vi "mod_Burst Detector.vi"(0 "IQ data (complex) in":cluster{"t0":dbl, "dt":dbl, "Y":cdb[]}={"t0"=0.0, "dt"=1.0, "Y"=[]} {"Y" format="%.2f"; "dt" format="%.2f"; "t0" format="%.2f"}, 1 "RC":dbl=0.001, 5 "Rise Trigger Specs":T2, 7 "Fall Trigger Specs":T1, 9 "Detection":enum16{"Simple", "Advanced"}(ring), 11 "error in (no error)":errorcluster, 12 "SC":dbl=0.0002, 13 "reset ? (T)":bool) -> (4 "Signal Envelope":waveform(dbl)(graph), 6 "Bursts Detected?":bool, 8 "Bursts Found":cluster{"Start Index":dbl, "Stop Index":dbl}[](array[cluster]), 10 "Number of Bursts":i32, 15 "error out":errorcluster)   [LabVIEW 2020, in "niDMT.lvlib"]
doc: "This utility detects multiple bursts. You can adjust the Discharge Time Constant (RC) and Charge Time Constant (SC) for detecting burst with short dead time between them. A lower value of RC implies fast discharging. For bursts very closely space, the discharging in the burst detector should happen fast so that falling slope is detected. Similarly SC can adjusted to detect rising between closely spaced bursts. Typically, the default values should work fine."
uses:
  <vilib>/addons/Modulation/niDMT.lvlib
  <vilib>/Analysis/baseanly.llb/Mean (DBL).vi
  <vilib>/measure/mamon.llb/Trigger Detection for 1 Channel (obs).vi
  <vilib>/Waveform/WDTOps.llb/WDT Get Waveform Subset DBL (LV80).vi
  <vilib>/addons/Modulation/niAMT.lvlib
  <vilib>/Analysis/NI_AALBase.lvlib
  <vilib>/measure/NI_MAPro.lvlib
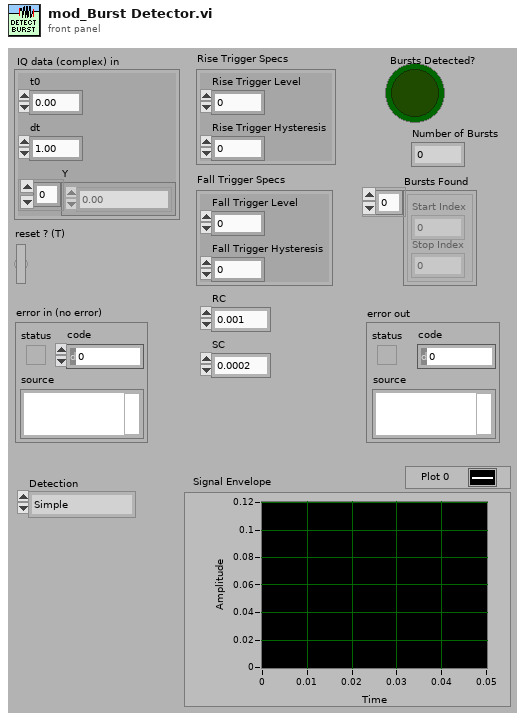
[diagram p1: front panel]
types:
  T1 = cluster{"Fall Trigger Level":dbl, "Fall Trigger Hysteresis":dbl}
  T2 = cluster{"Rise Trigger Level":dbl, "Rise Trigger Hysteresis":dbl}
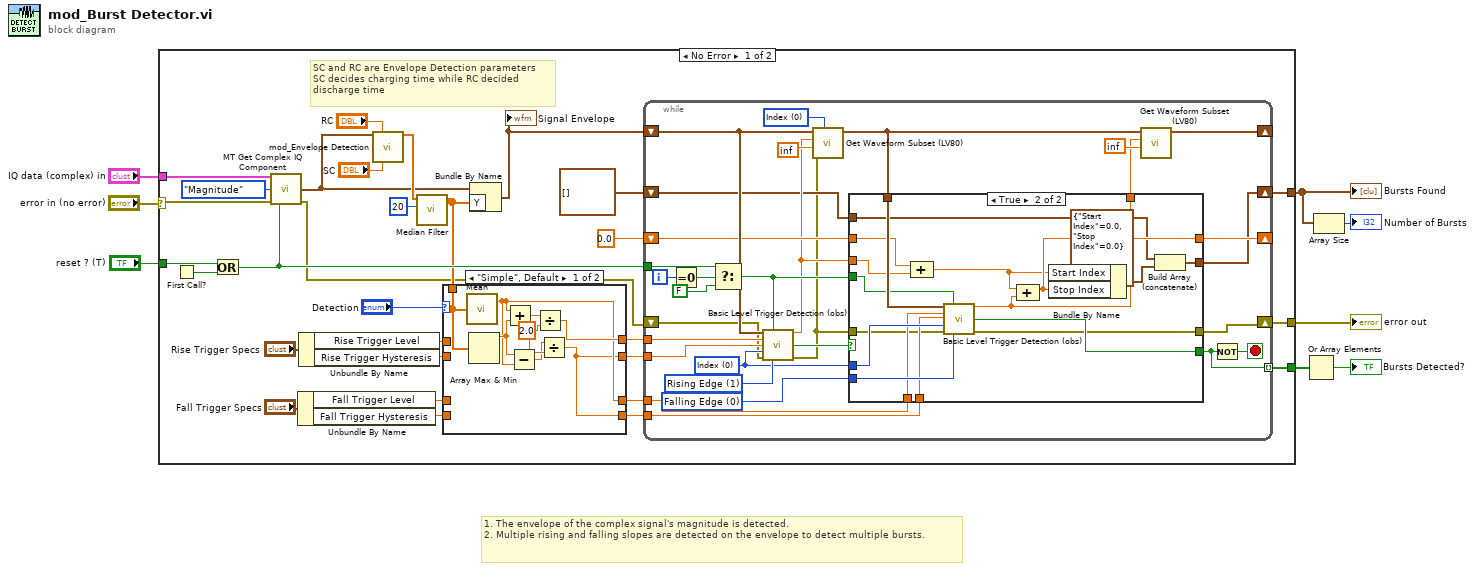
[diagram p0: block diagram]
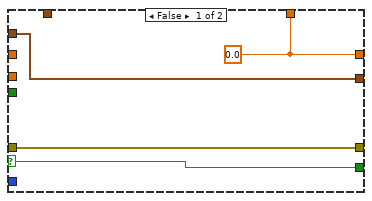
[diagram p3: hidden frame]
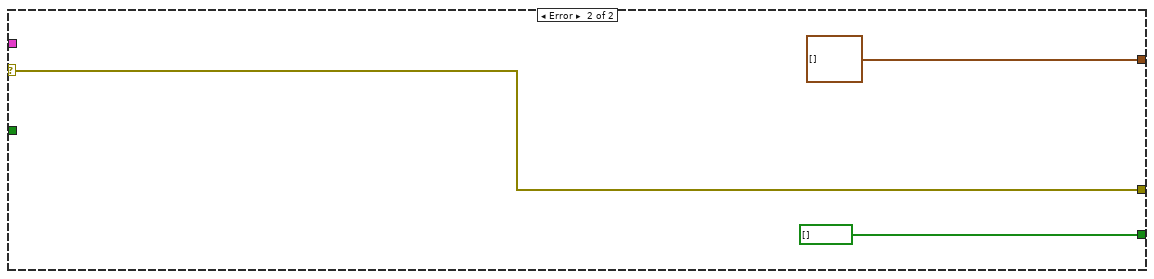
[diagram p4: hidden frame]
diagram:
  # "1. The envelope of the complex signal's magnitude is detected. \n2. Multiple rising and falling slopes are detected on the envelope to detect multiple bursts."
  n1 = case shown="No Error" "error in (no error)" {
    selector: "error in (no error)" -> [w37 w105]
    tunnel: "IQ data (complex) in" -> [w38 _]
    tunnel: "reset ? (T)" -> [w34 _]
    tunnel: [w24 cluster{"Start Index":dbl, "Stop Index":dbl}[] []] -> w2
    tunnel: [w22 bool[] []] -> w5
    tunnel: [w21 w105] -> w3
    frame No Error {
      # "SC and RC are Envelope Detection parameters\nSC decides charging time while RC decided \ndischarge time"
      n2 = First Call?() -> (First Call?: T/F=w35:bool)
      n3 = Or(x=w34, y=w35) -> (x .or. y?=w28:bool)
      n4 = call <vilib>:"MT Get Complex IQ Component.vi"("IQ data (complex) in"=w38, "reset? (F)"=w28, "component choice"=enum16{"I", "Q", "Magnitude", "Phase"}."Magnitude", "error in (no error)"=w37) -> ("CE component"=w29:waveform(dbl), "error out"=w9:errorcluster)  [unwired: 10 out]
      n5 = Unbundle By Name("Fall Trigger Specs") -> ("Fall Trigger Level"=w13:dbl, "Fall Trigger Hysteresis"=w11:dbl)
      n6 = Unbundle By Name("Rise Trigger Specs") -> ("Rise Trigger Level"=w15:dbl, "Rise Trigger Hysteresis"=w14:dbl)
      n7 = call <vilib>:"mod_Envelope Detection.vi"("input data"=w29, "RC"="RC", "SC"="SC") -> ("QP Output"=w31:dbl[])  [unwired: 12 out]
      n8 = call <vilib>:"Median Filter.vi"("left rank"=20 ("rank"), "X"=w31) -> ("Filtered X"=w19:dbl[])  [unwired: 1 in, 8 out]
      n9 = case shown="\"Simple\", Default" "Detection" {
        tunnel: w19 -> [w46 _]
        tunnel: [w40 w48] -> w18
        tunnel: [w39 w49] -> w17
        tunnel: [w44 w50] -> w16
        tunnel: w15 -> [_ w50]
        tunnel: w14 -> [_ w49]
        tunnel: w13 -> [_ w48]
        tunnel: [w39 w47] -> w12
        tunnel: w11 -> [_ w47]
        frame "Simple", Default {
          w42 = 2.0 ("y")
          n10 = call-poly <vilib>:"Mean.vi"("X"=w46) -> ("mean"=w40:dbl)  [unwired: 1 out]
          n11 = Array Max & Min(array=w46) -> (max value=w43:dbl)  [unwired: 3 out]
          n12 = Add(x=w40, y=w43) -> (x+y=w45:dbl)
          n13 = Subtract(x=w43, y=w40) -> (x-y=w41:dbl)
          n14 = Divide(x=w45, y=w42) -> (x/y=w44:dbl)
          n15 = Divide(x=w41, y=w42) -> (x/y=w39:dbl)
        }
        frame "Advanced" {
        }
      }
      n16 = Bundle By Name(cluster=w29, "Y"=w19) -> (w20:waveform(dbl))
      "Signal Envelope" <- w20
      n17 = while {
        shift-right: [w60] -> _
        shift-left: w20 -> [w72]
        tunnel: w28 -> [w78]
        tunnel: w16 -> [w77]
        tunnel: w17 -> [w76]
        tunnel: w18 -> [w68]
        tunnel: w12 -> [w67]
        shift-right: [w59] -> _
        shift-left: 0.0 -> [w62]
        shift-right: [w58] -> w24
        shift-left: cluster{"Start Index":dbl, "Stop Index":dbl}[] [] -> [w57]
        tunnel: [w55] -> w22 mode=indexing
        shift-right: [w51] -> w21
        shift-left: w9 -> [w53]
        i -> [w80]
        stop <- w56 stop-if-true
        w66 = u16 0 items=["Index", "Relative Time"] ("Mode")
        w69 = u16 0 items=["Falling Edge", "Rising Edge"] ("slope")
        w75 = u16 1 items=["Falling Edge", "Rising Edge"] ("slope")
        w70 = u16 0 items=["Index", "Time"] ("mode")
        n18 = Equal To 0?(x=w80) -> (x = 0?=w79:bool)
        n19 = Select(t=w78, s=w79, f=FALSE) -> (s? t:f=w71:bool)
        n20 = call-poly <vilib>:"Basic Level Trigger Detection (obs).vi"("signal in"=w72, "reset"=w71, "level"=w77, "hysteresis"=w76, "location mode"=w70, "error in (no error)"=w53, "trigger slope"=w75) -> ("trigger location"=w61:dbl, "trigger detected?"=w74:bool, "error out"=w52:errorcluster)  [unwired: 6 out]
        n21 = call-poly <vilib>:"Get Waveform Subset (LV80).vi"("start/duration format"=w66, "error in (no error)"=w52, "duration"=inf, "start samples/time"=w61, "waveform in"=w72) -> ("waveform out"=w64:waveform(dbl))  [unwired: 4 out]
        n22 = case shown="True" w74 {
          selector: w74 -> [w83 _]
          tunnel: w64 -> [_ w102]
          tunnel: w71 -> [_ w90]
          tunnel: w70 -> [_ w101]
          tunnel: w69 -> [_ w100]
          tunnel: w68 -> [_ w99]
          tunnel: w67 -> [_ w98]
          tunnel: [w84 w97] -> w63
          tunnel: w62 -> [_ w88]
          tunnel: w61 -> [_ w89]
          tunnel: [w84 w95] -> w59
          tunnel: [w82 w93] -> w58
          tunnel: w57 -> [w82 w92]
          tunnel: [w83 w91] -> w55
          tunnel: w52 -> [w81 w87]
          tunnel: [w81 w86] -> w51
          frame False {
            w84 = 0.0
          }
          frame True {
            n23 = Compound Arithmetic op=ADD(w88, w89) -> (w85:dbl)
            n24 = call-poly <vilib>:"Basic Level Trigger Detection (obs).vi"("signal in"=w102, "reset"=w90, "level"=w99, "hysteresis"=w98, "location mode"=w101, "error in (no error)"=w87, "trigger slope"=w100) -> ("trigger location"=w97:dbl, "trigger detected?"=w91:bool, "error out"=w86:errorcluster)  [unwired: 6 out]
            n25 = Compound Arithmetic op=ADD(w85, w97) -> (w95:dbl)
            n26 = Bundle By Name(cluster=cluster{"Start Index":dbl, "Stop Index":dbl} {"Start Index"=0.0, "Stop Index"=0.0}, "Start Index"=w85, "Stop Index"=w95) -> (w94:cluster{"Start Index":dbl, "Stop Index":dbl})
            n27 = Build Array (concatenate)(w92, w94) -> (w93:cluster{"Start Index":dbl, "Stop Index":dbl}[])
          }
        }
        n28 = call-poly <vilib>:"Get Waveform Subset (LV80).vi"("duration"=inf, "start samples/time"=w63, "waveform in"=w64) -> ("waveform out"=w60:waveform(dbl))  [unwired: 2 in, 4 out]
        n29 = Not(x=w55) -> (.not. x?=w56:bool)
      }
    }
    frame Error {
    }
  }
  "Bursts Found" <- w2
  "error out" <- w3
  n30 = Or Array Elements(Boolean array=w5) -> (logical OR=→"Bursts Detected?":bool)
  n31 = Array Size(array=w2) -> (size(s)=→"Number of Bursts":i32)
